vi "Query Remote Sense Calculation Status.vi"(8 "error in (no error)":errorcluster, 11 "VISA resource name":refnum<visa-resource-name>) -> (0 "error out":errorcluster, 2 "Calculation Status":i32(ring) items=["Dormant", "Calculating", "Complete"], 3 "VISA resource name out":refnum<visa-resource-name>)   [LabVIEW 2018, in "XP Power PLS600.lvlib"]
doc: "Queries the Remote Sense calculation status."
uses:
  XP Power PLS600.lvlib
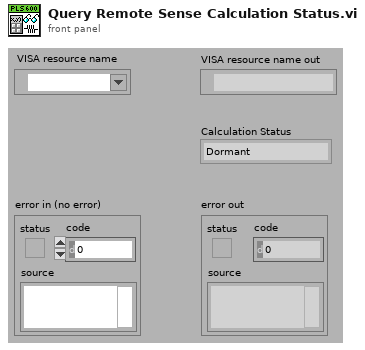
[diagram p1: front panel]
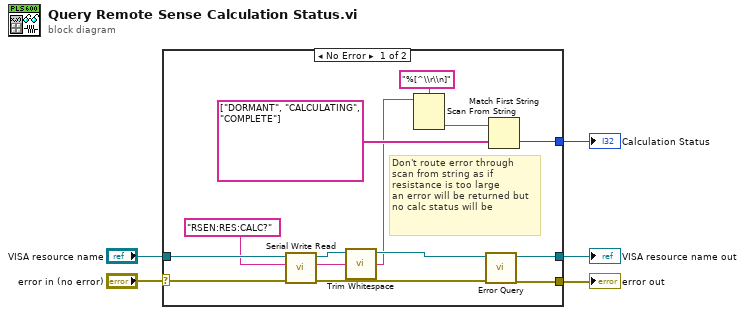
[diagram p0: block diagram]
diagram:
  n1 = case shown="No Error" "error in (no error)" {
    selector: "error in (no error)" -> [w9 w20]
    tunnel: [w18 w19] -> w5
    tunnel: [w17 w20] -> w4
    tunnel: [w15 _] -> w3
    tunnel: "VISA resource name" -> [w12 w19]
    frame No Error {
      # "Don't route error through\nscan from string as if\nresistance is too large\nan error will be returned but\nno calc status will be"
      n2 = call "Serial Write Read.vi"("error in (no error)"=w9, "Write Buffer"="RSEN:RES:CALC?", "VISA resource name"=w12) -> ("error out"=w6:errorcluster, "Read Buffer"=w8:string, "VISA resource name out"=w10:refnum<visa-resource-name>)  [unwired: 6 in]
      n3 = call <vilib>:"Trim Whitespace.vi"("string"=w8) -> ("trimmed string"=w7:string)  [unwired: 1 in]
      n4 = Scan From String(format string="%[^\\r\\n]", input string=w7) -> (output 1=w13:string)  [unwired: 3 in, 3 out]
      n5 = call "Error Query.vi"("error in (no error)"=w6, "VISA resource name"=w10) -> ("error out"=w17:errorcluster, "VISA resource name out"=w18:refnum<visa-resource-name>)  [unwired: 6 in, 2 out]
      n6 = Match First String(2:string[] ["DORMANT", "CALCULATING", "COMPLETE"], 3:w13) -> (0:w15:i32)  [unwired: 1 out]
    }
    frame Error {
    }
  }
  "Calculation Status" <- w3
  "VISA resource name out" <- w5
  "error out" <- w4
